vi "Exam.vi"() -> ()   [LabVIEW 2017]
panel:
  out "Phase 5":bool
  out "Phase 4":bool
  in  "Name":string
  in  "Path":path
  out "Phase 3":bool
  out "Phase 2":bool
  out "Phase 1":bool
  in  "Config":bool
  out "Waveform Graph":dbl[](graph)
  in  "Sample Rate":dbl
  in  "Boolean":bool
  in  "Frequency":dbl
  in  "T":dbl
  in  "Amplitude":dbl
  in  "stop":bool
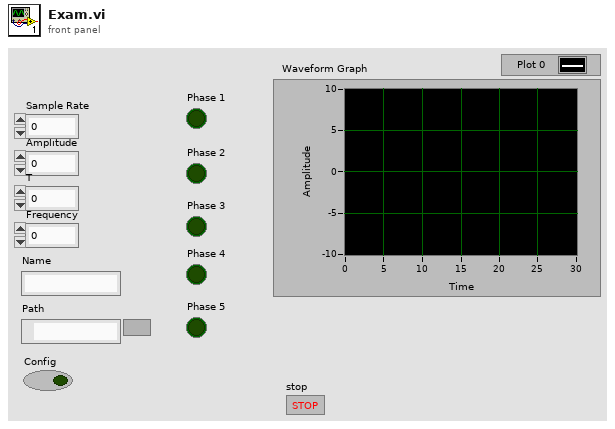
[diagram p1: front panel]
types:
  T1 = enum8{"Enabled", "Disabled", "Disabled and Grayed Out"}
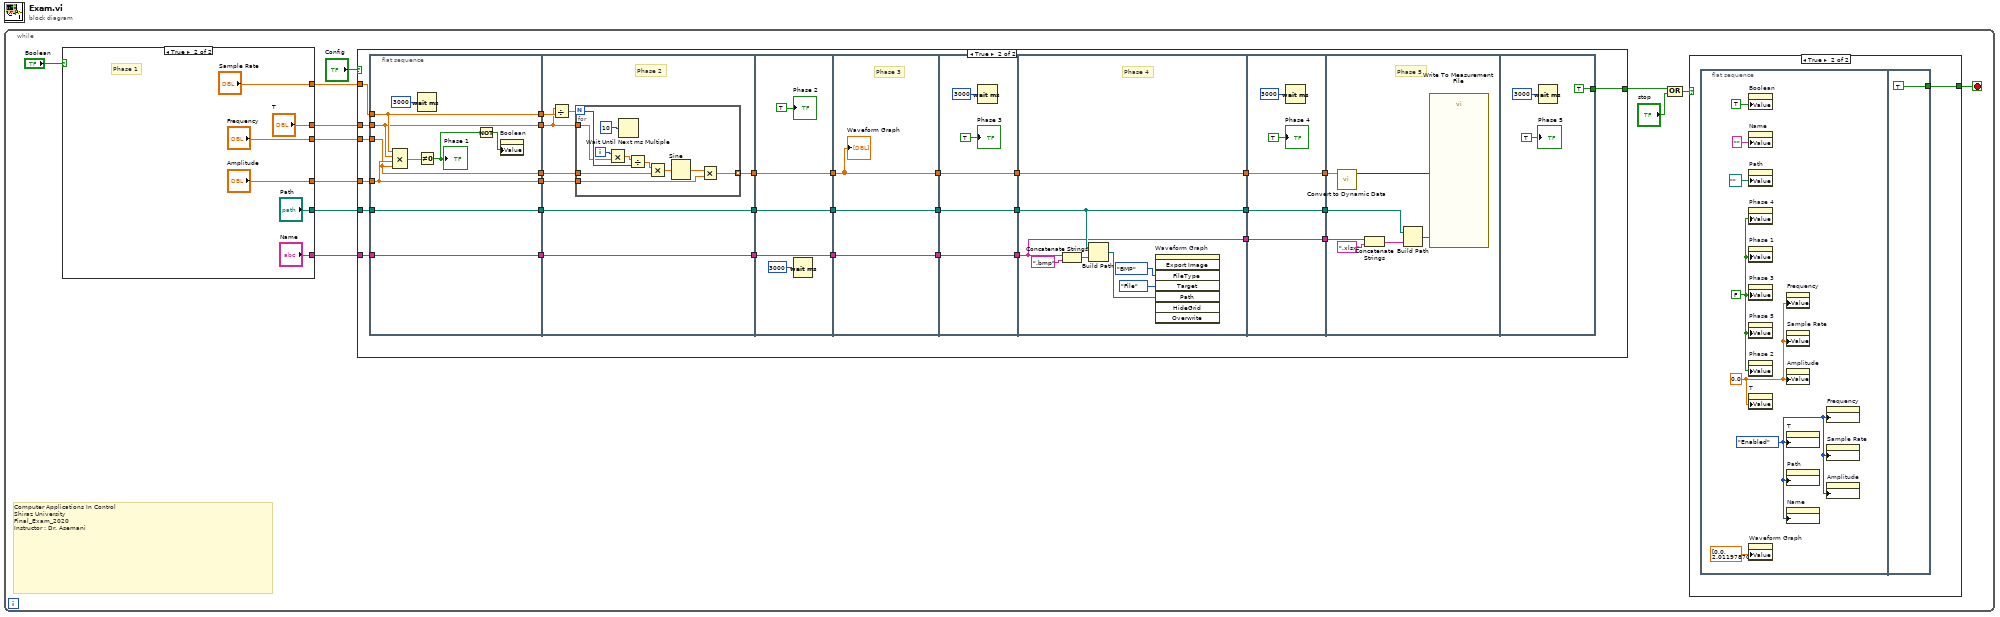
[diagram p0: block diagram]
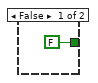
[diagram p2: hidden frame]
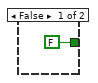
[diagram p3: hidden frame]
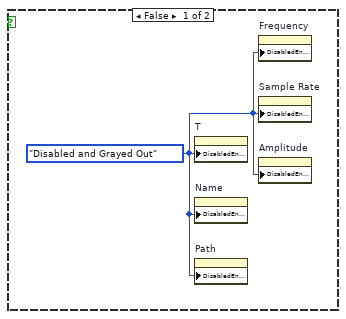
[diagram p4: hidden frame]
diagram:
  n1 = while {
    stop <- w8 stop-if-true
    # "Computer Applications In Control\nShiraz University\nFinal_Exam_2020\nInstructor : Dr. Asemani"
    n2 = case shown="True" "Boolean" {
      tunnel: [_ "Amplitude"] -> w12
      tunnel: [_ "T"] -> w11
      tunnel: [_ "Frequency"] -> w10
      tunnel: [_ "Sample Rate"] -> w5
      tunnel: [_ "Path"] -> w2
      tunnel: [_ "Name"] -> w1
      frame False {
        w120 = T1."Disabled and Grayed Out" ("Disabled")
        n3 = property on="T" class="DigNum (strict)"("DisabledEnum"=w120) -> ()  [unwired: 2 in, 2 out]
        n4 = property on="Name" class="Str"("DisabledEnum"=w120) -> ()  [unwired: 2 in, 2 out]
        n5 = property on="Path" class="Path"("DisabledEnum"=w120) -> ()  [unwired: 2 in, 2 out]
        n6 = property on="Frequency" class="DigNum (strict)"("DisabledEnum"=w120) -> ()  [unwired: 2 in, 2 out]
        n7 = property on="Sample Rate" class="DigNum (strict)"("DisabledEnum"=w120) -> ()  [unwired: 2 in, 2 out]
        n8 = property on="Amplitude" class="DigNum (strict)"("DisabledEnum"=w120) -> ()  [unwired: 2 in, 2 out]
      }
      frame True {
        # "Phase 1"
      }
    }
    n9 = case shown="True" "Config" {
      tunnel: w12 -> [_ w54]
      tunnel: w11 -> [_ w53]
      tunnel: w10 -> [_ w52]
      tunnel: w5 -> [_ w51]
      tunnel: [FALSE ("Phase 2") w40] -> w3
      tunnel: w2 -> [_ w34]
      tunnel: w1 -> [_ w28]
      frame False {
      }
      frame True {
        n10 = flat-sequence {
          tunnel: w51 -> [w64]
          tunnel: w52 -> [w61]
          tunnel: w53 -> [w63]
          tunnel: w54 -> [w62]
          tunnel: [w62] -> w50
          tunnel: [w63] -> w49
          tunnel: [w61] -> w48
          tunnel: [w64] -> w47
          tunnel: [w56] -> w35
          tunnel: w34 -> [w56]
          tunnel: [w55] -> w29
          tunnel: w28 -> [w55]
          tunnel: w50 -> [w69]
          tunnel: w49 -> [w68]
          tunnel: w48 -> [w70]
          tunnel: w47 -> [w72]
          tunnel: [w67] -> w45
          tunnel: [w66] -> w36
          tunnel: w35 -> [w66]
          tunnel: [w65] -> w30
          tunnel: w29 -> [w65]
          tunnel: [w88] -> w46
          tunnel: w45 -> [w88]
          tunnel: [w85] -> w37
          tunnel: w36 -> [w85]
          tunnel: [w84] -> w31
          tunnel: w30 -> [w84]
          tunnel: w46 -> [w91]
          tunnel: [w91] -> w43
          tunnel: [w90] -> w38
          tunnel: w37 -> [w90]
          tunnel: [w89] -> w32
          tunnel: w31 -> [w89]
          tunnel: [w94] -> w44
          tunnel: w43 -> [w94]
          tunnel: [w93] -> w39
          tunnel: w38 -> [w93]
          tunnel: [w92] -> w33
          tunnel: w32 -> [w92]
          tunnel: w44 -> [w104]
          tunnel: [w104] -> w41
          tunnel: w39 -> [w100]
          tunnel: w33 -> [w98]
          tunnel: [w100] -> w27
          tunnel: [w98] -> w24
          tunnel: [w107] -> w42
          tunnel: w41 -> [w107]
          tunnel: w27 -> [w106]
          tunnel: [w106] -> w26
          tunnel: [w105] -> w25
          tunnel: w24 -> [w105]
          tunnel: w42 -> [w116]
          tunnel: w26 -> [w113]
          tunnel: w25 -> [w111]
          tunnel: [TRUE ("Phase 2")] -> w40
          frame #0 {
            n11 = Compound Arithmetic op=MULTIPLY(w64, w63, w62, w61) -> (w60:dbl)
            n12 = Wait (ms)(milliseconds to wait=u32 3000) -> ()  [unwired: 1 out]
            n13 = Not Equal To 0?(x=w60) -> (x != 0?=w59:bool)
            "Phase 1" <- w59
            n14 = Not(x=w59) -> (.not. x?=w58:bool)
            n15 = property on="Boolean" class="Bool (strict)"("Value"=w58) -> ()  [unwired: 2 in, 2 out]
          }
          frame #1 {
            # "Phase 2"
            n16 = Divide(x=w68, y=w72) -> (x/y=w71:dbl)
            n17 = for {
              N: w71 -> [w82]
              tunnel: w70 -> [w77]
              tunnel: [w78] -> w67 mode=indexing
              tunnel: w69 -> [w79]
              tunnel: w68 -> [w74]
              i -> [w75]
              n18 = Multiply(x=w75, y=w74) -> (x*y=w83:dbl)
              n19 = Wait Until Next ms Multiple(millisecond multiple=u32 10) -> ()  [unwired: 1 out]
              n20 = Divide(x=w83, y=w82) -> (x/y=w76:dbl)
              n21 = Multiply(x=w76, y=w77) -> (x*y=w81:dbl)
              n22 = Sine(x=w81) -> (sin(x)=w80:dbl)
              n23 = Multiply(x=w80, y=w79) -> (x*y=w78:dbl)
            }
          }
          frame #2 {
            n24 = Wait (ms)(milliseconds to wait=u32 3000) -> ()  [unwired: 1 out]
            "Phase 2" <- TRUE ("Phase 2")
          }
          frame #3 {
            # "Phase 3"
            "Waveform Graph" <- w91
          }
          frame #4 {
            n25 = Wait (ms)(milliseconds to wait=u32 3000) -> ()  [unwired: 1 out]
            "Phase 3" <- TRUE ("Phase 2")
          }
          frame #5 {
            # "Phase 4"
            n26 = Concatenate Strings(w98, ".bmp" ("string")) -> (w99:string)
            n27 = Build Path(base path=w100, name or relative path=w99) -> (appended path=w101:path)
            n28 = invoke on="Waveform Graph" class="WFGraph (strict)" method="Export Image"("FileType"=enum32{"BMP", "EPS", "EMF", "PICT"}."BMP" ("File Type"), "Target"=enum32{"File", "Clipboard"}."File", "Path"=w101) -> ()  [unwired: 5 in, 8 out]
          }
          frame #6 {
            n29 = Wait (ms)(milliseconds to wait=u32 3000) -> ()  [unwired: 1 out]
            "Phase 4" <- TRUE ("Phase 2")
          }
          frame #7 {
            # "Phase 5"
            n30 = call "Convert to Dynamic Data"("Array"=w116) -> ("Dynamic Data Type"=w115:dynamicdata)  [unwired: 3 in]
            n31 = Concatenate Strings(w111, ".xlsx" ("string")) -> (w112:string)
            n32 = Build Path(base path=w113, name or relative path=w112) -> (appended path=w114:path)
            n33 = call "Write To Measurement File"("Signals"=w115, "Filename"=w114) -> ()  [unwired: 15 in, 3 out]
          }
          frame #8 {
            n34 = Wait (ms)(milliseconds to wait=u32 3000) -> ()  [unwired: 1 out]
            "Phase 5" <- TRUE ("Phase 2")
          }
        }
      }
    }
    n35 = Compound Arithmetic op=OR(w3, "stop") -> (w7:bool)
    n36 = case shown="True" w7 {
      tunnel: [FALSE w14] -> w8
      frame False {
      }
      frame True {
        n37 = flat-sequence {
          tunnel: [TRUE] -> w14
          frame #0 {
            w18 = FALSE ("Boolean")
            w20 = 0.0 ("Numeric")
            w15 = T1."Enabled" ("Disabled")
            n38 = property on="Boolean" class="Bool (strict)"("Value"=TRUE ("Boolean")) -> ()  [unwired: 2 in, 2 out]
            n39 = property on="Name" class="Str"("Value"="" ("Name")) -> ()  [unwired: 2 in, 2 out]
            n40 = property on="Path" class="Path"("Value"=path "" ("Path")) -> ()  [unwired: 2 in, 2 out]
            n41 = property on="Phase 4" class="Bool (strict)"("Value"=w18) -> ()  [unwired: 2 in, 2 out]
            n42 = property on="Phase 1" class="Bool (strict)"("Value"=w18) -> ()  [unwired: 2 in, 2 out]
            n43 = property on="Phase 3" class="Bool (strict)"("Value"=w18) -> ()  [unwired: 2 in, 2 out]
            n44 = property on="Phase 5" class="Bool (strict)"("Value"=w18) -> ()  [unwired: 2 in, 2 out]
            n45 = property on="Phase 2" class="Bool (strict)"("Value"=w18) -> ()  [unwired: 2 in, 2 out]
            n46 = property on="T" class="DigNum (strict)"("Value"=w20) -> ()  [unwired: 2 in, 2 out]
            n47 = property on="Waveform Graph" class="WFGraph (strict)"("Value"=dbl[] [0.0, 2.0119787051797875, 3.9416699756714726, 5.7101518308497194, 7.245095555315886, 8.483723853688193, 9.375378364154585, 9.883591522667064, 9.987578041100525, 9.683084999768493, 8.982565786565718, 7.914670768842408, 6.523075528898921, 4.86469458681657, 3.0073536671461527, 1.0270157108608806, -0.9953259147542701, -2.9769599444128323, -4.836840003035663, -6.498899302014303, -7.895161676561143, -8.968521726575684, -9.675080356712137, -9.985940194955083, -9.888387459309358, -9.386411935721723, -8.50054380078196, -7.267013962952707, -5.736272263330623, -3.970924139690845, -2.0431701416971313] ("Waveform Graph")) -> ()  [unwired: 2 in, 2 out]
            n48 = property on="Frequency" class="DigNum (strict)"("Value"=w20) -> ()  [unwired: 2 in, 2 out]
            n49 = property on="Sample Rate" class="DigNum (strict)"("Value"=w20) -> ()  [unwired: 2 in, 2 out]
            n50 = property on="Amplitude" class="DigNum (strict)"("Value"=w20) -> ()  [unwired: 2 in, 2 out]
            n51 = property on="T" class="DigNum (strict)"("DisabledEnum"=w15) -> ()  [unwired: 2 in, 2 out]
            n52 = property on="Path" class="Path"("DisabledEnum"=w15) -> ()  [unwired: 2 in, 2 out]
            n53 = property on="Name" class="Str"("DisabledEnum"=w15) -> ()  [unwired: 2 in, 2 out]
            n54 = property on="Frequency" class="DigNum (strict)"("DisabledEnum"=w15) -> ()  [unwired: 2 in, 2 out]
            n55 = property on="Sample Rate" class="DigNum (strict)"("DisabledEnum"=w15) -> ()  [unwired: 2 in, 2 out]
            n56 = property on="Amplitude" class="DigNum (strict)"("DisabledEnum"=w15) -> ()  [unwired: 2 in, 2 out]
          }
          frame #1 {
          }
        }
      }
    }
  }
